vi "Untitled 2.vi"() -> ()   [LabVIEW 2017]
panel:
  out "Right":dbl
  out "Left":dbl
  in  "XAxis":dbl
  in  "YAxis":dbl
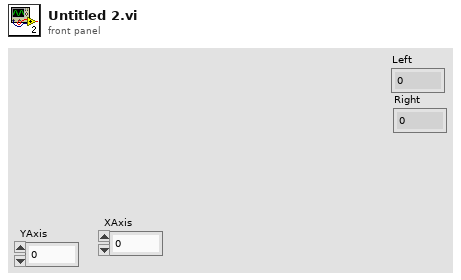
[diagram p1: front panel]
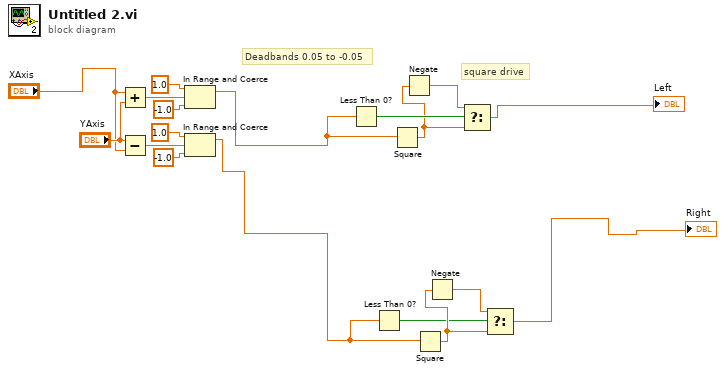
[diagram p0: block diagram]
diagram:
  # "square drive"
  # "Deadbands 0.05 to -0.05"
  n1 = Add(x="XAxis", y="YAxis") -> (x+y=w17:dbl)
  n2 = Subtract(x="YAxis", y="XAxis") -> (x-y=w12:dbl)
  n3 = In Range and Coerce(upper limit=1.0, x=w17, lower limit=-1.0) -> (coerced(x)=w9:dbl)  [unwired: 1 out]
  n4 = In Range and Coerce(upper limit=1.0, x=w12, lower limit=-1.0) -> (coerced(x)=w3:dbl)  [unwired: 1 out]
  n5 = Less Than 0?(x=w9) -> (x < 0?=w11:bool)
  n6 = Less Than 0?(x=w3) -> (x < 0?=w4:bool)
  n7 = Square(x=w9) -> (x^2=w8:dbl)
  n8 = Negate(x=w8) -> (-x=w10:dbl)
  n9 = Square(x=w3) -> (x^2=w6:dbl)
  n10 = Negate(x=w6) -> (-x=w5:dbl)
  n11 = Select(t=w10, s=w11, f=w8) -> (s? t:f=→"Left":dbl)
  n12 = Select(t=w5, s=w4, f=w6) -> (s? t:f=→"Right":dbl)
